vi "GenerateCode.vi"(0 "XRef":T10, 1 "Terms":T7, 2 "Diagram":T6, 3 "State In":T1) -> (14 "Generated Code?":T5, 15 "Reply":T3, 16 "Fatal Error Out":T2, 17 "State Out":T1)   [LabVIEW 2015, in "LVJSON.lvlib" / "Get Object Parameters.xnode"]
uses:
  Get Object Parameters.xnode
  <vilib>/XNodeSupport/XNodeXNodeRef.ctl
  <vilib>/XNodeSupport/XNodeTermIDPairs.ctl
  <vilib>/XNodeSupport/XNodeTermIDPair.ctl
  <vilib>/XNodeSupport/XNodeTermRef.ctl
  <vilib>/XNodeSupport/XNodeString.ctl
  <vilib>/XNodeSupport/XNodeTopLevelDiagramRef.ctl
  State.ctl
  <vilib>/XNodeSupport/XNodeBool.ctl
  <vilib>/XNodeSupport/XNodeStringArray.ctl
  <vilib>/XNodeSupport/XNodeErrorCluster.ctl
  <vilib>/Utility/miscctls.llb/LVPointTypeDef.ctl
  Get Parameter Value.vi
  <vilib>/XNodeSupport/NI_XNodeSupport.lvlib
  JSON Object.lvclass
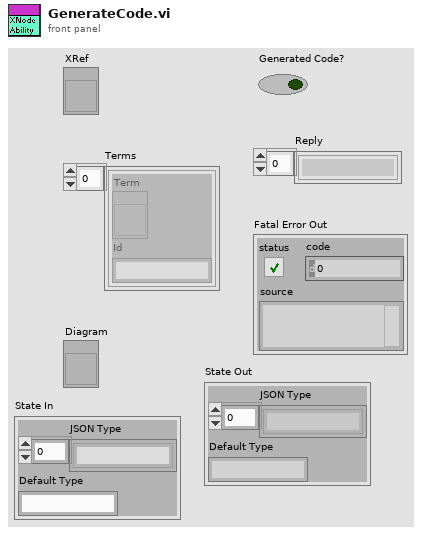
[diagram p1: front panel]
types:
  T1 = typedef "LVJSON.lvlib/Get Object Parameters.xnode/State.ctl" = cluster{"JSON Type":string[], "Default Type":string}
  T2 = typedef "NI_XNodeSupport.lvlib/XNodeErrorCluster.ctl" = errorcluster
  T3 = typedef "NI_XNodeSupport.lvlib/XNodeStringArray.ctl" = T4[]
  T4 = typedef "NI_XNodeSupport.lvlib/XNodeString.ctl" = string
  T5 = typedef "NI_XNodeSupport.lvlib/XNodeBool.ctl" = bool
  T6 = typedef "NI_XNodeSupport.lvlib/XNodeTopLevelDiagramRef.ctl" = refnum<vi>
  T7 = typedef "NI_XNodeSupport.lvlib/XNodeTermIDPairs.ctl" = T8[]
  T8 = typedef "NI_XNodeSupport.lvlib/XNodeTermIDPair.ctl" = cluster{"Term":T9, "Id":T4}
  T9 = typedef "NI_XNodeSupport.lvlib/XNodeTermRef.ctl" = refnum<vi>
  T10 = typedef "NI_XNodeSupport.lvlib/XNodeXNodeRef.ctl" = refnum<vi>
  T11 = typedef "LVPointTypeDef.ctl" = cluster{"Horizontal":i16, "Vertical":i16}
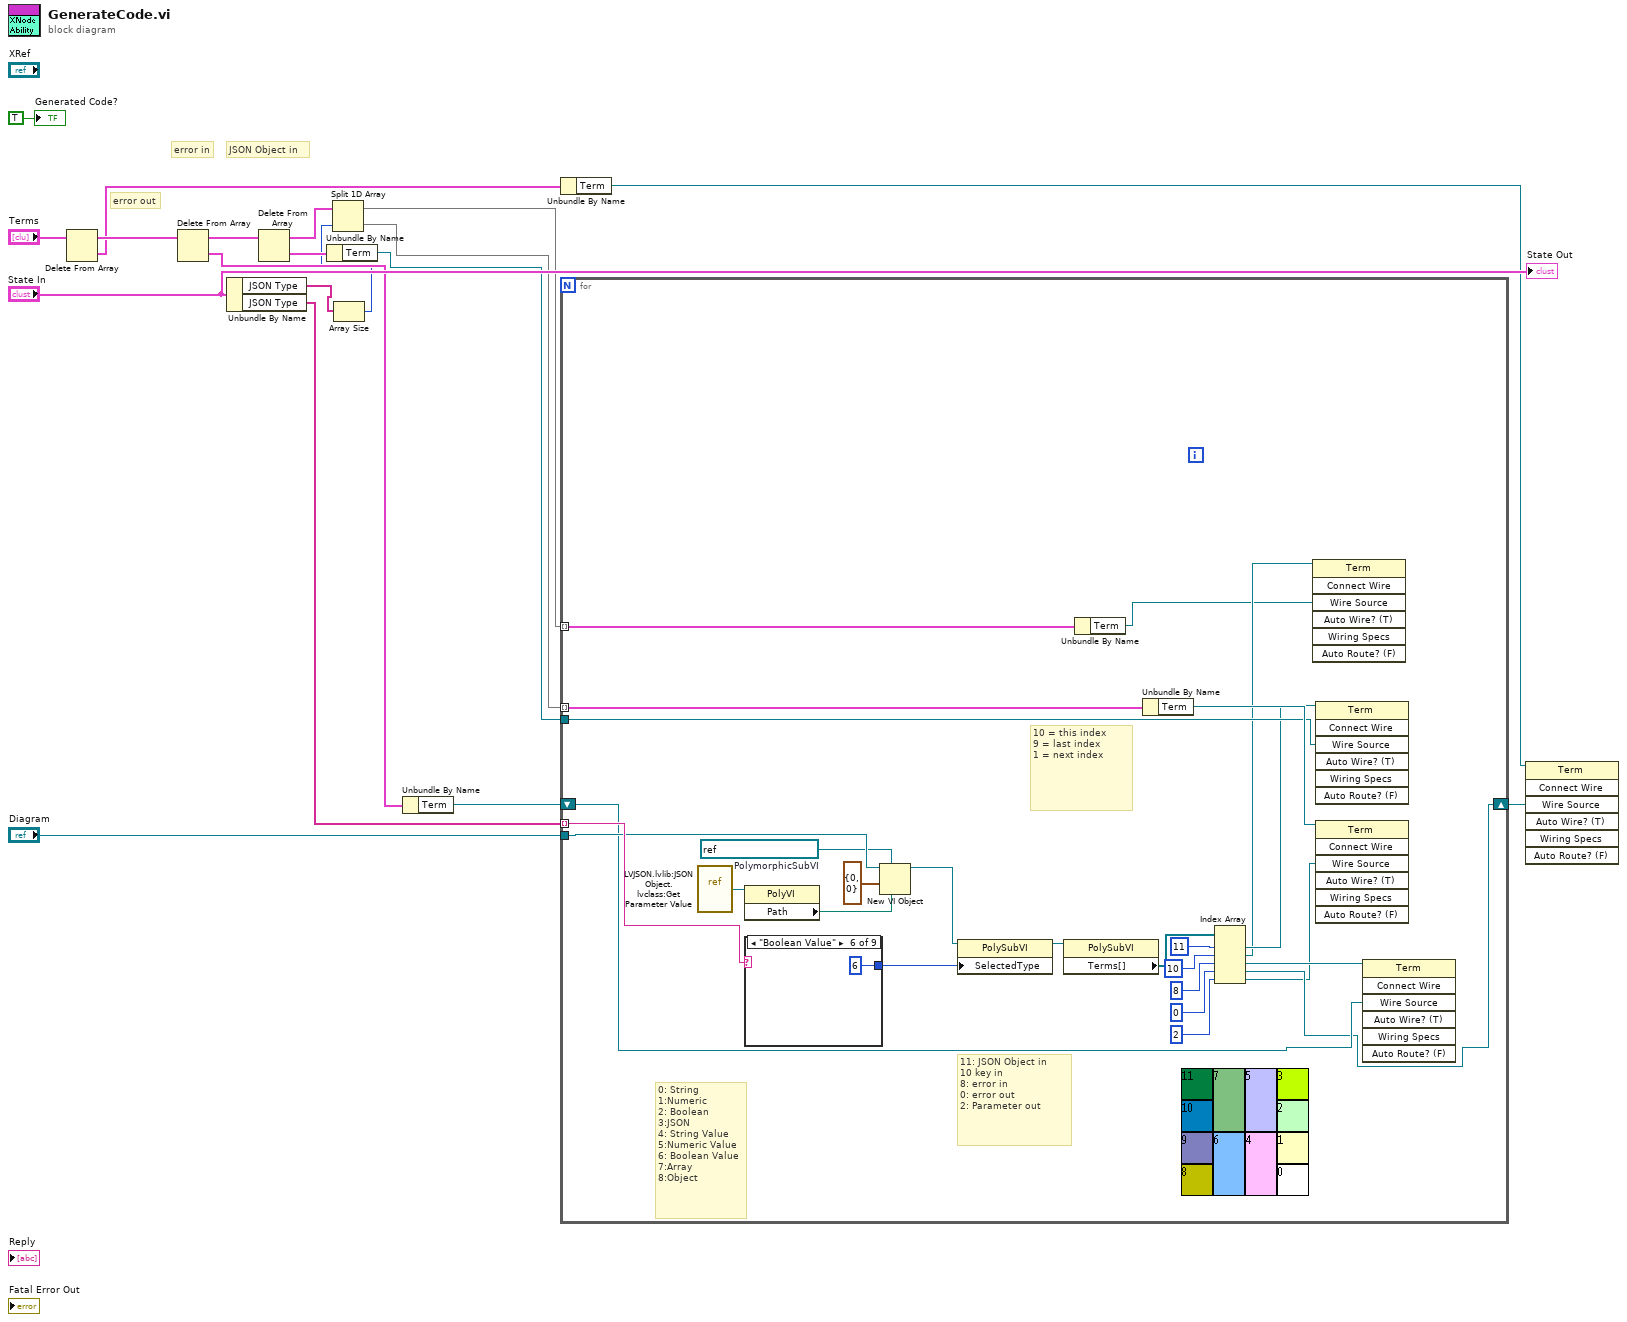
[diagram p0: block diagram]
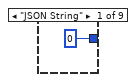
[diagram p2: hidden frame]
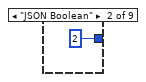
[diagram p3: hidden frame]
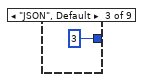
[diagram p4: hidden frame]
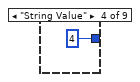
[diagram p5: hidden frame]
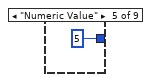
[diagram p6: hidden frame]
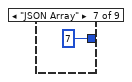
[diagram p7: hidden frame]
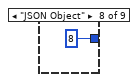
[diagram p8: hidden frame]
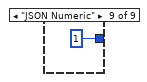
[diagram p9: hidden frame]
diagram:
  # "JSON Object in"
  # "error in"
  # "error out"
  n1 = Delete From Array(array="Terms") -> (deleted portion=w7:T8, array with subset deleted=w9:T7)  [unwired: 2 in]
  n2 = Delete From Array(array=w9) -> (deleted portion=w6:T8, array with subset deleted=w8:T7)  [unwired: 2 in]
  n3 = Unbundle By Name("State In") -> ("JSON Type"=w2:string[], "JSON Type"=w11:string[])
  n4 = Delete From Array(array=w8) -> (deleted portion=w13:T8, array with subset deleted=w14:T7)  [unwired: 2 in]
  n5 = Unbundle By Name(w13) -> ("Term"=w12:T9)
  n6 = Array Size(array=w2) -> (size(s)=w1:i32)
  n7 = Split 1D Array(array=w14, index=w1) -> (first subarray=w17:T7, second subarray=w16:T7)
  n8 = Unbundle By Name(w6) -> ("Term"=w5:T9)
  n9 = Unbundle By Name(w7) -> ("Term"=w4:T9)
  n10 = for {
    tunnel: w17 -> [w44] mode=indexing
    tunnel: w16 -> [w45] mode=indexing
    tunnel: "Diagram" -> [w40]
    tunnel: w12 -> [w38]
    tunnel: w11 -> [w43] mode=indexing
    shift-right: [w23] -> w3
    shift-left: w5 -> [w39]
    w33 = refnum<vi> refnum  # PolymorphicSubVI
    # "0: String\n1:Numeric\n2: Boolean\n3:JSON\n4: String Value\n5:Numeric Value\n6: Boolean Value\n7:Array\n8:Object"
    # "11: JSON Object in\n10 key in\n8: error in\n0: error out\n2: Parameter out"
    # "10 = this index\n9 = last index\n1 = next index"
    n11 = vi-ref "LVJSON.lvlib:JSON Object.lvclass:Get Parameter Value.vi"() -> (w30:refnum<vi>)
    n12 = property class="PolyVI"(reference=w30) -> ("Path"=w32:path)  [unwired: 1 in, 2 out]
    n13 = case shown="\"Boolean Value\"" w43 {
      tunnel: [0 ("Selected Type") 2 ("Selected Type") 3 ("Selected Type") 4 ("Selected Type") 5 ("Selected Type") 6 ("Selected Type") 7 ("Selected Type") 8 ("Selected Type") 1 ("Selected Type")] -> w41
      frame "JSON String" {
      }
      frame "JSON Boolean" {
      }
      frame "JSON", Default {
      }
      frame "String Value" {
      }
      frame "Numeric Value" {
      }
      frame "Boolean Value" {
      }
      frame "JSON Array" {
      }
      frame "JSON Object" {
      }
      frame "JSON Numeric" {
      }
    }
    n14 = New VI Object(vi object class=w33, owner refnum=w40, position/next to=T11 {"Horizontal"=0, "Vertical"=0} ("location"), 6:w32) -> (object refnum=w31:refnum<vi>)  [unwired: 4 in, 1 out]
    n15 = property class="PolySubVI"(reference=w31, "SelectedType"=w41) -> (reference out=w35:refnum<vi>)  [unwired: 1 in, 1 out]
    n16 = property class="PolySubVI"(reference=w35) -> ("Terms[]"=w36:refnum<vi>[])  [unwired: 1 in, 2 out]
    n17 = Unbundle By Name(w44) -> ("Term"=w20:T9)
    n18 = Unbundle By Name(w45) -> ("Term"=w42:T9)
    n19 = Index Array(array=w36, index #1=11 ("index"), index #2=10 ("index"), index #3=8 ("index"), index #4=0 ("index"), index #5=2 ("index")) -> (element #1=w28:refnum<vi>, element #2=w21:refnum<vi>, element #3=w25:refnum<vi>, element #4=w23:refnum<vi>, element #5=w22:refnum<vi>)
    n20 = invoke class="Term" method="Connect Wire"(reference=w21, "Wire Source"=w20) -> ()  [unwired: 5 in, 7 out]
    n21 = invoke class="Term" method="Connect Wire"(reference=w28, "Wire Source"=w38) -> ()  [unwired: 5 in, 7 out]
    n22 = invoke class="Term" method="Connect Wire"(reference=w42, "Wire Source"=w22) -> ()  [unwired: 5 in, 7 out]
    n23 = invoke class="Term" method="Connect Wire"(reference=w25, "Wire Source"=w39) -> ()  [unwired: 5 in, 7 out]
  }
  n24 = invoke class="Term" method="Connect Wire"(reference=w4, "Wire Source"=w3) -> ()  [unwired: 5 in, 7 out]
  "Generated Code?" <- T5 TRUE ("Generated Code?")
  "State Out" <- "State In"
